vi "INIT.vi"(0 "VISA resource name":refnum<visa-resource-name>="GPIB0::24::INSTR", 11 "error in (no error)":errorcluster) -> (4 "VISA resource name out":refnum<visa-resource-name>, 15 "error out":errorcluster)   [LabVIEW 2010]
doc: "INITiate\n:INITiate[:IMMediate] Take SourceMeter out of idle state.\nDescription This command is used to initiate source-measure operation by taking the SourceMeter out of idle. The :READ? and :MEASure? commands also perform an initiation.\n\nNote that if auto output-off is disabled (SOURce1:CLEar:AUTO OFF), the source output must first be turned on before an initiation can be performed.\nThe :MEASure? command automatically turns the output source on before performing the initiation."
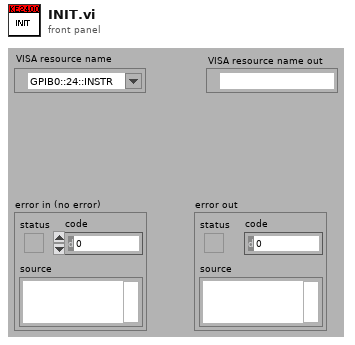
[diagram p1: front panel]
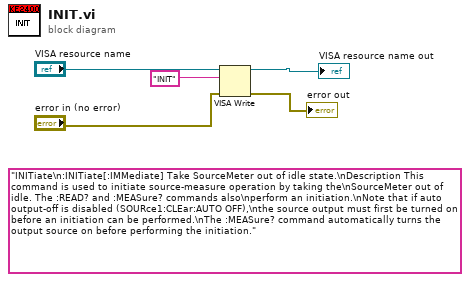
[diagram p0: block diagram]
diagram:
  (unwired) "INITiate\n:INITiate[:IMMediate] Take SourceMeter out of idle state.\nDescription This command is used to initiate source-measure operation by taking the\nSourceMeter out of idle. The :READ? and :MEASure? commands also\nperform an initiation.\nNote that if auto output-off is disabled (SOURce1:CLEar:AUTO OFF),\nthe source output must first be turned on before an initiation can be performed.\nThe :MEASure? command automatically turns the output source on before performing the initiation."
  n1 = VISA Write(VISA resource name="VISA resource name", write buffer="INIT", error in (no error)="error in (no error)") -> (VISA resource name out=→"VISA resource name out":refnum<visa-resource-name>, error out=→"error out":errorcluster)  [unwired: 1 out]
